vi "Get Paths.vi"(8 "error in (no error)":errorcluster, 11 "ParseXML in":refnum<class "ParseSVG.lvclass">) -> (0 "error out":errorcluster, 3 "ParseXML out":refnum<class "ParseSVG.lvclass">)   [LabVIEW 2019, in "ParseSVG.lvclass"]
uses:
  ParseSVG.lvclass
  Path.ctl
  ParseSVG.lvclass/ParseSVG.ctl
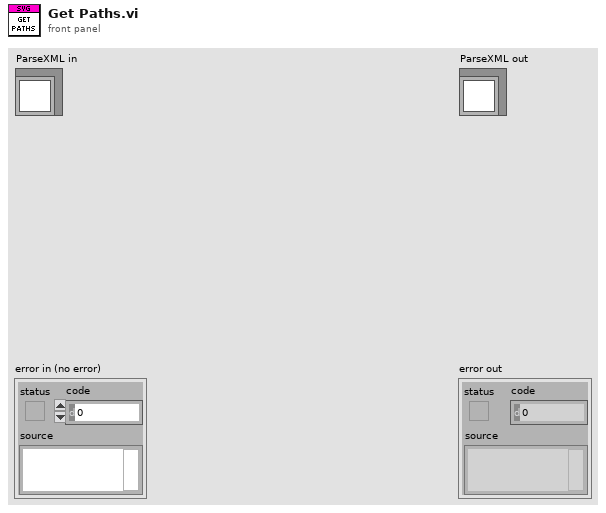
[diagram p1: front panel]
types:
  T1 = typedef "ParseSVG.lvclass/Path.ctl" = cluster{"d":string, "style":string, "transform":string}
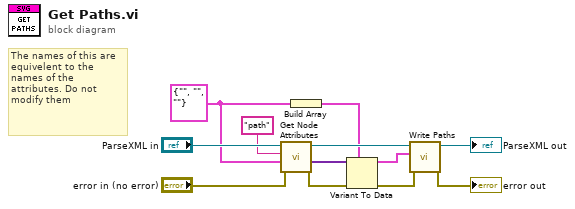
[diagram p0: block diagram]
diagram:
  w1 = T1 {"d"="", "style"="", "transform"=""} ("Path")
  # "The names of this are equivelent to the names of the attributes. Do not modify them"
  n1 = call "Get Node Attributes.vi"("error in (no error)"="error in (no error)", "Attributes Cluster"=w1, "Node Name (exact)"="path", "ParseSVG in"="ParseXML in") -> ("error out"=w6:errorcluster, "[Attributes Cluster]"=w7:variant[], "ParseSVG out"=w10:refnum<class "ParseSVG.lvclass">)  [unwired: 5 in]
  n2 = Build Array(w1) -> (w8:T1[])
  n3 = Variant To Data(error in=w6, type=w8, Variant=w7) -> (data=w5:T1[], error out=w3:errorcluster)
  n4 = call "Write Paths.vi"("error in (no error)"=w3, "Paths"=w5, "ParseXML in"=w10) -> ("error out"=→"error out":errorcluster, "ParseXML out"=→"ParseXML out":refnum<class "ParseSVG.lvclass">)  [unwired: 7 in]
